vi "Update_c.vi"(7 "Reset":bool=TRUE, 8 "input valid":bool=TRUE, 10 "delta_c":fxp<+/-,32,4>) -> (0 "output valid":bool, 3 "c out":fxp<+/-,32,4>)   [LabVIEW 2013]
doc: "Increases Fi with Fi_delta. Also wraps Fi to the range [0, 2*Pi]"
uses:
  <vilib>/rvi/FXPMathLib/FxpAdd/XNode/nifxpmath_Add.xnode
  <vilib>/rvi/FXPMathLib/sim/FxpSim.dll
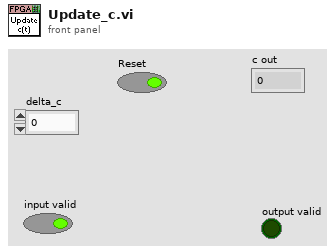
[diagram p1: front panel]
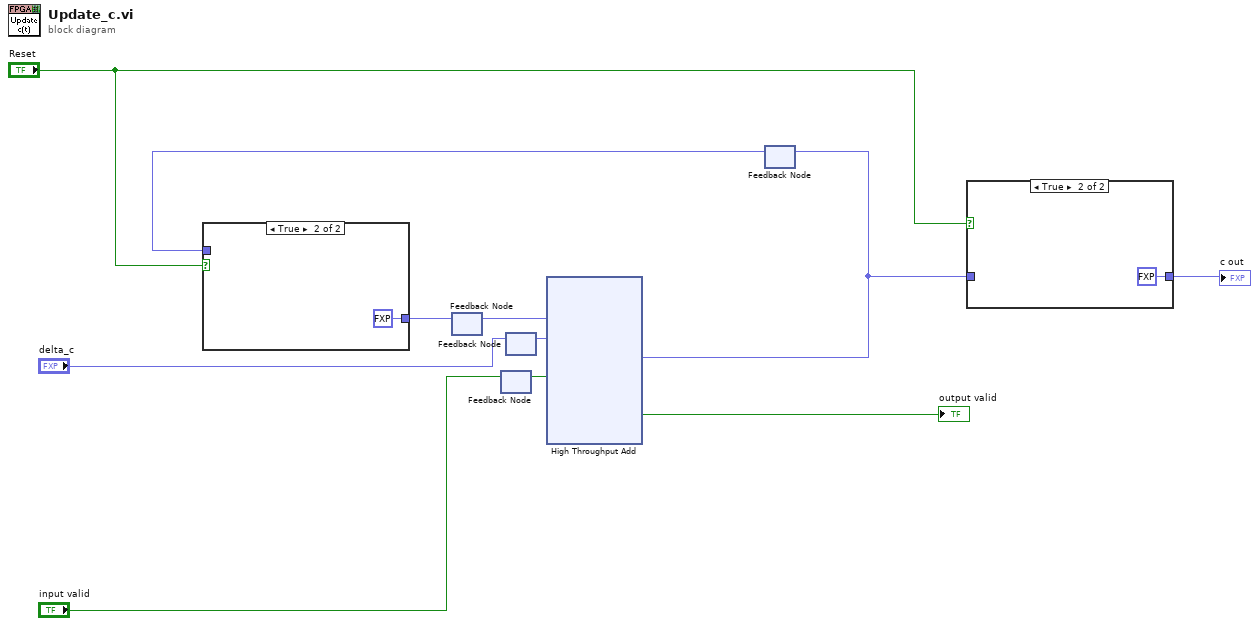
[diagram p0: block diagram]
diagram:
  n1 = feedback #1() -> (w10:fxp<+/-,32,4>)  [unwired: 1 in]
  n2 = feedback #2() -> (w7:bool)  [unwired: 1 in]
  n3 = feedback-in #2("input valid") -> ()
  n4 = feedback #3() -> (w9:fxp<+/-,32,4>)  [unwired: 1 in]
  n5 = feedback-in #3("delta_c") -> ()
  n6 = xnode "High Throughput Add"("x"=w10, "y"=w9, "input valid"=w7) -> ("x+y"=w2:fxp<+/-,32,4>, "output valid"=→"output valid":bool)  [unwired: 1 in, 1 out]
  n7 = feedback-in #4(w2) -> ()
  n8 = feedback #4() -> (w6:fxp<+/-,32,4>)  [unwired: 1 in]
  n9 = case shown="True" "Reset" {
    tunnel: [w12 fxp<+/-,32,4> 0.0 ("x_out")] -> w11
    tunnel: w6 -> [w12 _]
    frame False {
    }
    frame True {
    }
  }
  n10 = feedback-in #1(w11) -> ()
  n11 = case shown="True" "Reset" {
    tunnel: [w14 fxp<+/-,32,4> 0.0 ("x_out")] -> w1
    tunnel: w2 -> [w14 _]
    frame False {
    }
    frame True {
    }
  }
  "c out" <- w1
